vi "ExpandTree.vi"(8 "error in (no error)":errorcluster, 10 "ToExpand in":refnum<data-value>, 11 "SudukuBoard in":refnum<class "SudukuBoard.lvclass">) -> (0 "error out":errorcluster, 1 "ExpandedSearchNodes":refnum<data-value>[](array[refnum]), 2 "ToExpand out":refnum<data-value>, 3 "SudukuBoard out":refnum<class "SudukuBoard.lvclass">)   [LabVIEW 2009, in "SudukuBoard.lvclass"]
uses:
  SudukuBoard.lvclass
  SudukuState/SudukuState.lvclass
  EXPANDmethod.ctl
  TreeNode/TreeNode.lvclass
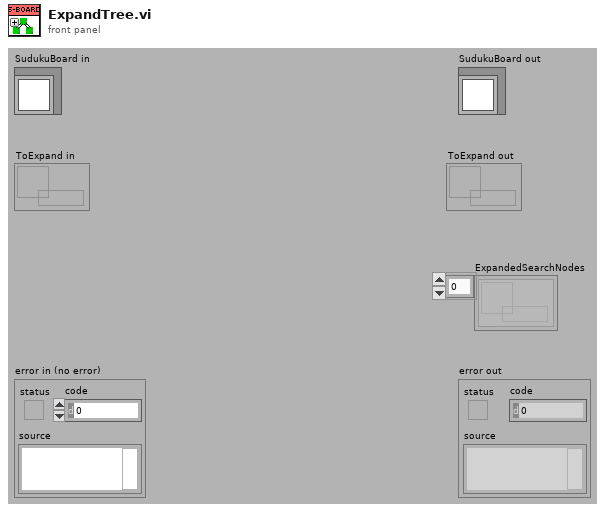
[diagram p1: front panel]
types:
  T1 = typedef "SudukuBoard.lvclass/EXPANDmethod.ctl" = enum16{"shotgun", "row", "column", "number"}
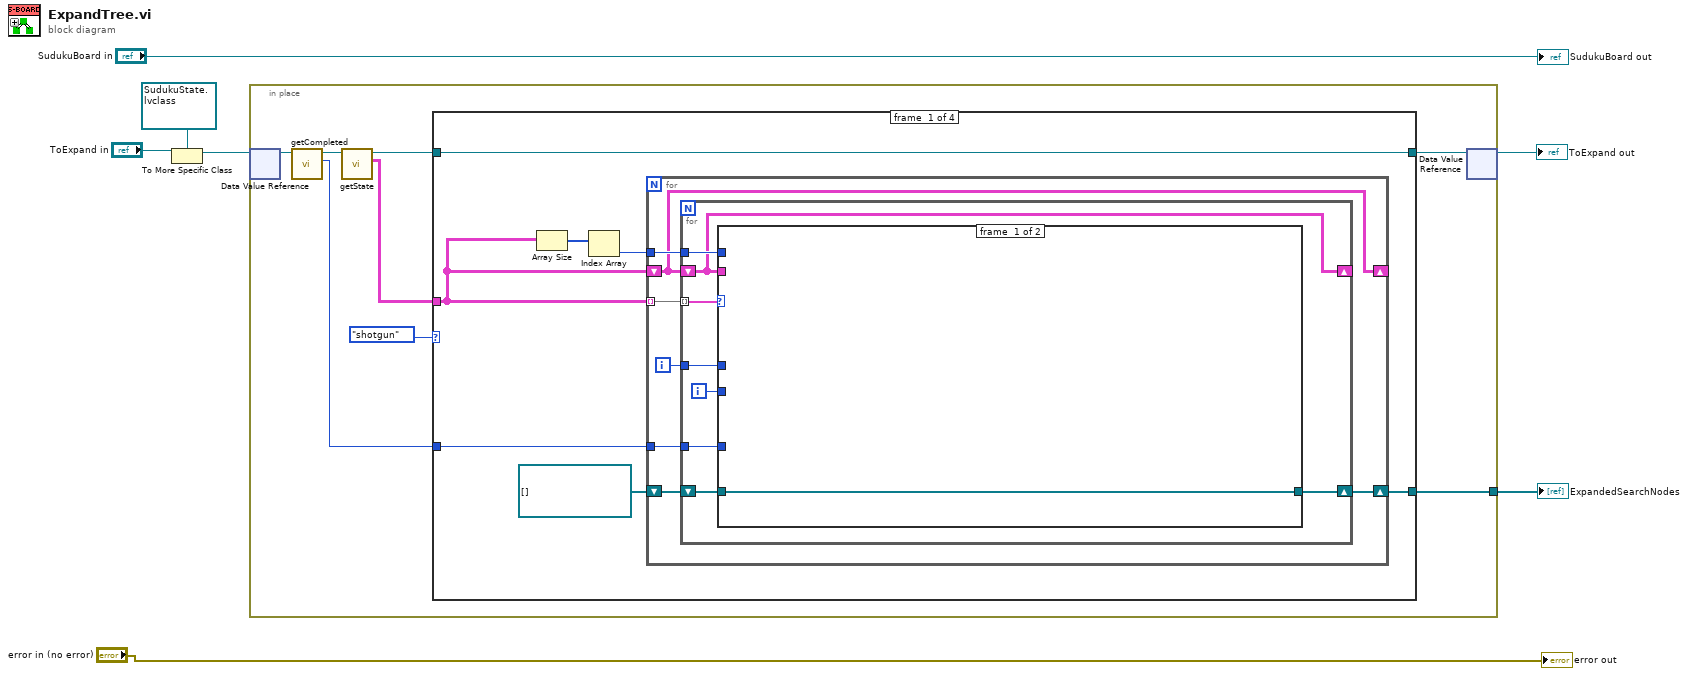
[diagram p0: block diagram]
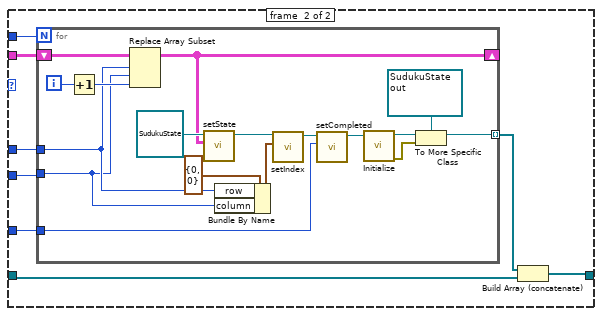
[diagram p2: hidden frame]
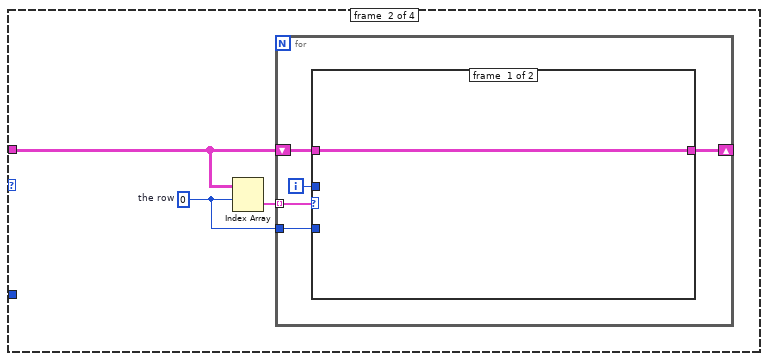
[diagram p3: hidden frame]
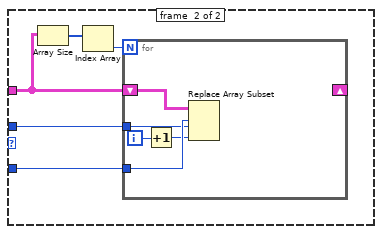
[diagram p4: hidden frame]
diagram:
  n1 = To More Specific Class(target class=refnum<data-value> refnum ("data value reference"), reference="ToExpand in") -> (specific class reference=w6:refnum<data-value>)  [unwired: 1 in, 1 out]
  n2 = in-place {
    in-place-border: [w14] -> w3
    n3 = in-place-dvr #1(w6) -> (w13:refnum<class "SudukuState.lvclass">)  [unwired: 1 out]
    n4 = call "getCompleted.vi"("SudukuState in"=w13) -> ("completed"=w11:i32, "SudukuState out"=w12:refnum<class "SudukuState.lvclass">)  [unwired: 8 in, 1 out]
    n5 = call "getState.vi"("SudukuState in"=w12) -> ("State"=w15:cluster{"Value":i32, "Options":i32[]}[][], "SudukuState out"=w10:refnum<class "SudukuState.lvclass">)  [unwired: 8 in, 1 out]
    n6 = case shown="\"row\"" EXPANDmethod."shotgun" ("EXPAND") {
      tunnel: w15 -> [w22 w66 _ _]
      tunnel: [w18 _ _ _] -> w14
      tunnel: w11 -> [w17 _ _ _]
      tunnel: w10 -> [w16 _ _ _]
      tunnel: [w16 _ _ _] -> w9
      frame #0 {
        n7 = Array Size(array=w22) -> (size(s)=w21:i32[])
        n8 = Index Array(array=w21) -> (element=w20:i32)  [unwired: 1 in]
        n9 = for {
          tunnel: w22 -> [w29] mode=indexing
          shift-right: [w26] -> _
          shift-left: w22 -> [w26]
          tunnel: w20 -> [w28]
          shift-right: [w24] -> w18
          shift-left: refnum<data-value>[] [] -> [w25]
          tunnel: w17 -> [w23]
          i -> [w27]
          n10 = for {
            tunnel: w29 -> [w37] mode=indexing
            tunnel: w28 -> [w36]
            shift-right: [w33] -> _
            shift-left: w26 -> [w33]
            tunnel: w27 -> [w35]
            shift-right: [w31] -> w24
            shift-left: w25 -> [w32]
            tunnel: w23 -> [w30]
            i -> [w34]
            n11 = case shown="0" w37 {
              tunnel: w36 -> [_ w46]
              tunnel: w33 -> [_ w45]
              tunnel: w35 -> [_ w44]
              tunnel: w34 -> [_ w43]
              tunnel: w32 -> [w38 w40]
              tunnel: [w38 w41] -> w31
              tunnel: w30 -> [_ w39]
              frame #0 {
              }
              frame #1 {
                n12 = for {
                  N: w46 -> [_]
                  shift-right: [w59] -> _
                  shift-left: w45 -> [w62]
                  tunnel: w44 -> [w52]
                  tunnel: w43 -> [w51]
                  tunnel: [w56] -> w42 mode=indexing
                  tunnel: w39 -> [w47]
                  i -> [w63]
                  n13 = Increment(x=w63) -> (x+1=w61:i32)
                  n14 = Replace Array Subset(array=w62, new element=w61, index (row)=w52, index (col)=w51) -> (w59:cluster{"Value":i32, "Options":i32[]}[][])
                  n15 = call "setState.vi"("State"=w59, "SudukuState in"=refnum<class "SudukuState.lvclass"> refnum ("SudukuState.lvclass")) -> ("SudukuState out"=w54:refnum<class "SudukuState.lvclass">)  [unwired: 8 in, 1 out]
                  n16 = Bundle By Name(cluster=cluster{"row":i32, "column":i32} {"row"=0, "column"=0} ("index"), "row"=w52, "column"=w51) -> (w50:cluster{"row":i32, "column":i32})
                  n17 = call "setIndex.vi"("index"=w50, "SudukuState in"=w54) -> ("SudukuState out"=w49:refnum<class "SudukuState.lvclass">)  [unwired: 8 in, 1 out]
                  n18 = call "setCompleted.vi"("completed"=w47, "SudukuState in"=w49) -> ("SudukuState out"=w48:refnum<class "SudukuState.lvclass">)  [unwired: 8 in, 1 out]
                  n19 = call-dynamic "Initialize.vi"("GraphNode data"=w48) -> ("error out"=w58:errorcluster, "Node out"=w57:refnum<data-value>)  [unwired: 9 in]
                  n20 = To More Specific Class(target class=refnum<data-value> refnum ("data value reference"), reference=w57, error in=w58) -> (specific class reference=w56:refnum<data-value>)  [unwired: 1 out]
                }
                n21 = Build Array (concatenate)(w42, w40) -> (w41:refnum<data-value>[])
              }
            }
          }
        }
      }
      frame #1 {
        w65 = 0  # the row
        n22 = Index Array(array=w66, index (row)=w65) -> (element=w64:cluster{"Value":i32, "Options":i32[]}[])  [unwired: 1 in]
        n23 = for {
          tunnel: w64 -> [w71] mode=indexing
          shift-right: [w69] -> _
          shift-left: w66 -> [w70]
          tunnel: w65 -> [w68]
          i -> [w67]
          n24 = case shown="0" w71 {
            tunnel: w70 -> [w72 w77]
            tunnel: [w72 _] -> w69
            tunnel: w68 -> [_ w74]
            tunnel: w67 -> [_ w73]
            frame #0 {
            }
            frame #1 {
              n25 = Array Size(array=w77) -> (size(s)=w76:i32[])
              n26 = Index Array(array=w76) -> (element=w75:i32)  [unwired: 1 in]
              n27 = for {
                N: w75 -> [_]
                shift-right: _ -> [_]
                shift-left: w77 -> [w82]
                tunnel: w74 -> [w81]
                tunnel: w73 -> [w78]
                i -> [w80]
                n28 = Increment(x=w80) -> (x+1=w79:i32)
                n29 = Replace Array Subset(array=w82, new element=w79, index (row)=w81, index (col)=w78) -> ()  [unwired: 1 out]
              }
            }
          }
        }
      }
      frame #2 {
      }
      frame #3 {
      }
    }
    n30 = in-place-dvr #1(w9) -> (→"ToExpand out":refnum<data-value>)  [unwired: 1 out]
  }
  "ExpandedSearchNodes" <- w3
  "error out" <- "error in (no error)"
  "SudukuBoard out" <- "SudukuBoard in"
